vi "generate_play.vi"(0 "task/channels in":refnum<k21>, 1 "error in":errorcluster) -> (2 "task out":refnum<k21>, 3 "task done?":bool, 4 "error out":errorcluster)   [LabVIEW 2017]
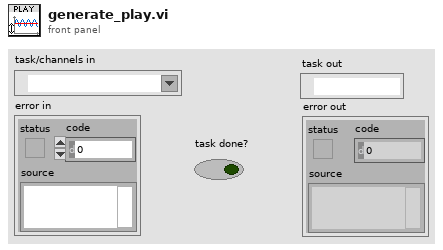
[diagram p1: front panel]
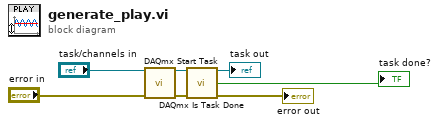
[diagram p0: block diagram]
diagram:
  n1 = call <vilib>:"DAQmx Start Task.vi"("task/channels in"="task/channels in", "error in"="error in") -> ("task out"=w7:refnum<k21>, "error out"=w6:errorcluster)  [unwired: 12 in]
  n2 = call <vilib>:"DAQmx Is Task Done.vi"("task/channels in"=w7, "error in"=w6) -> ("task out"=→"task out":refnum<k21>, "task done?"=→"task done?":bool, "error out"=→"error out":errorcluster)  [unwired: 11 in]
